vi "Circular Equal Division Points.vi"(6 "Para":T2, 8 "错误输入":errorcluster, 11 "Center":T1) -> (0 "错误输出":errorcluster, 2 "Relative Point Array":T1[](array[typedef]), 3 "Absolute Point Array":T1[](array[typedef]))   [LabVIEW 2012, in "Picture Box Tools.lvlib" / "Basic Shape.lvlib"]
uses:
  Basic Shape.lvlib
  Point Custom Control.ctl
  <vilib>/Analysis/1siggen.llb/Ramp Pattern by Samples.vi
  <vilib>/Analysis/NI_AALBase.lvlib
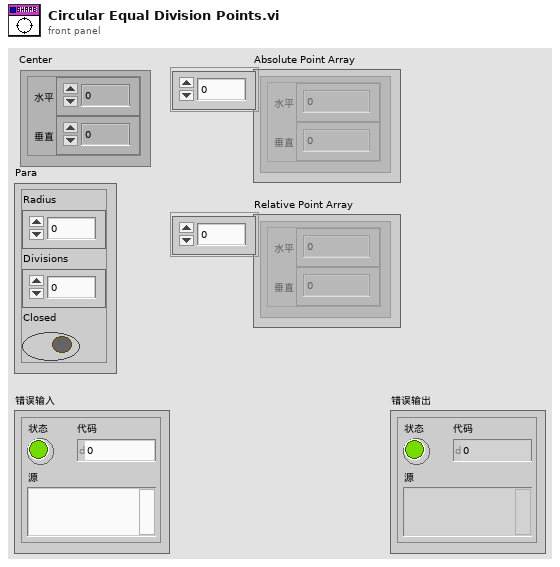
[diagram p1: front panel]
types:
  T1 = typedef "Picture Box Tools.lvlib/Basic Shape.lvlib/Point Custom Control.ctl" = cluster{"horizontal":i16, "vertical":i16}
  T2 = cluster{"Radius":i16, "Divisions":i16, "Closed":bool}
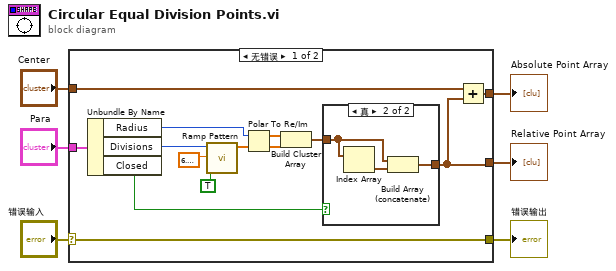
[diagram p0: block diagram]
diagram:
  n1 = case shown="无错误" "错误输入" {
    selector: "错误输入" -> [w20 w25]
    tunnel: [w20 w25] -> w5
    tunnel: "Para" -> [w19 _]
    tunnel: "Center" -> [w13 _]
    tunnel: [w12 _] -> w2
    tunnel: [w11 _] -> w1
    frame No Error {
      n2 = Unbundle By Name(w19) -> ("Radius"=w16:i16, "Divisions"=w18:i16, "Closed"=w15:bool)
      n3 = call-poly <vilib>:"Ramp Pattern.vi"("exclude end?"=TRUE, "end"=6.283185307179586, "samples"=w18) -> ("Ramp Pattern"=w17:dbl[])  [unwired: 7 in, 1 out]
      n4 = Polar To Re/Im(2:w17, 3:w16) -> (0:w9:dbl[], 1:w10:dbl[])
      n5 = Build Cluster Array(w10, w9) -> (w14:cluster{dbl, dbl}[])
      n6 = case shown="真" w15 {
        tunnel: w14 -> [w21 w24]
        tunnel: [w21 w22] -> w11
        frame False {
        }
        frame True {
          n7 = Index Array(array=w24) -> (element=w23:cluster{dbl, dbl})  [unwired: 1 in]
          n8 = Build Array (concatenate)(w24, w23) -> (w22:cluster{dbl, dbl}[])
        }
      }
      n9 = Add(x=w13, y=w11) -> (x+y=w12:cluster{dbl, dbl}[])
    }
    frame Error {
    }
  }
  "错误输出" <- w5
  "Absolute Point Array" <- w2
  "Relative Point Array" <- w1
